vi "serialization tests.vi"() -> ()   [LabVIEW 2013, in "TEC tests.lvlib"]
uses:
  TEC tests.lvlib
  <vilib>/NI/Tag Bus Module Framework/channel/channel classification.ctl
  configuration/TEC configuration.lvclass
  <vilib>/NI/Configuration Framework/serializable configuration/NISE_CEF_serializable configuration.lvclass/NISE_CEF_serializable configuration.ctl
  <vilib>/NI/Configuration Framework/serializable configuration/NISE_CEF_serializable configuration.lvclass
  configuration/TEC configuration.lvclass/TEC configuration.ctl
  <vilib>/NI/Configuration Framework/serializable configuration/Read UID.vi
  configuration/Write channels.vi
  configuration/Read channels.vi
  <vilib>/NI/Tag Bus Module Framework/channel/TBM channel.lvclass
panel:
  out "channels equal":bool
  out "no error":errorcluster
  out "no error":errorcluster
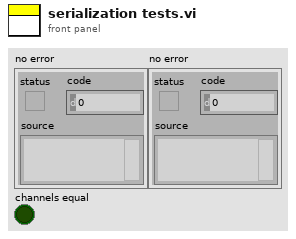
[diagram p1: front panel]
types:
  T1 = typedef "TBM channel.lvclass/channel classification.ctl" = enum16{"input data", "output data", "processing parameter", "processing result"}
  T2 = typedef "tag bus.lvlib/tag descriptor.lvclass/Data Type.ctl" = enum16{"Double", "Single", "I64", "I32", "I16", "I8", "U64", "U32", "U16", "U8", "Boolean", "String", "Array of Double", "Array of Single", "Array of I64", "Array of I32", "Array of I16", "Array of I8", "Array of U64", "Array of U32", "Array of U16", "Array of U8", "Array of Boolean", "Array of String"}
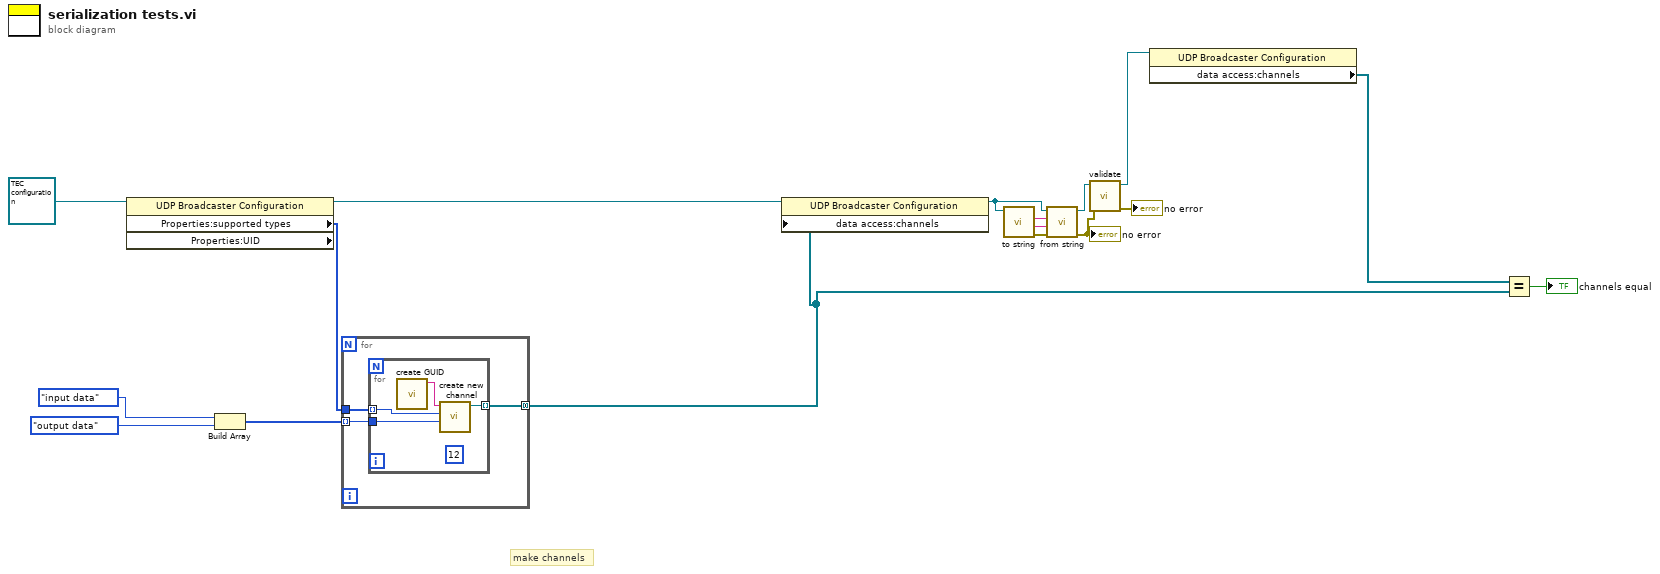
[diagram p0: block diagram]
diagram:
  # "make channels"
  n1 = property class="UDP Broadcaster Configuration" props=["Properties:supported types", "Properties:UID"](reference=refnum<class "TEC configuration.lvclass"> refnum ("tag bus configurable plugin module configuration")) -> (reference out=w5:refnum<class "TEC configuration.lvclass">, "Properties:supported types"=w9:T2[])  [unwired: 1 in, 2 out]
  n2 = Build Array(channel_classification."input data" ("channel classification"), channel_classification."output data" ("channel classification")) -> (w10:T1[])
  n3 = for {
    tunnel: w10 -> [w20] mode=indexing
    tunnel: [w19] -> w1 mode=concatenating
    tunnel: w9 -> [w18]
    n4 = for {
      tunnel: w20 -> [w23]
      tunnel: [w24] -> w19 mode=indexing
      tunnel: w18 -> [w22] mode=indexing
      (unwired) 12
      n5 = call <vilib>:"create GUID.vi"() -> ("uuid"=w21:string)  [unwired: 11 in]
      n6 = call <vilib>:"create new channel.vi"("channel classification"=w23, "data type"=w22, "channel name"=w21) -> ("channel"=w24:refnum<class "TBM channel.lvclass">)  [unwired: 8 in]
    }
  }
  n7 = property class="UDP Broadcaster Configuration"(reference=w5, "data access:channels"=w1) -> (reference out=w2:refnum<class "TEC configuration.lvclass">)  [unwired: 1 in, 1 out]
  n8 = call-dynamic "to string.vi"("TEC configuration in"=w2) -> ("error out"=w17:errorcluster, "data"=w16:string, "version"=w15:string)  [unwired: 7 in, 1 out]
  n9 = call-dynamic "from string.vi"("error in"=w17, "data"=w16, "version"=w15, "TEC configuration in"=w2) -> ("error out"=w8:errorcluster, "TEC configuration out"=w14:refnum<class "TEC configuration.lvclass">)  [unwired: 6 in]
  "no error" <- w8
  n10 = call-dynamic "validate.vi"("error in"=w8, "TEC configuration in"=w14) -> ("error out"=→"no error":errorcluster, "TEC configuration out"=w4:refnum<class "TEC configuration.lvclass">)  [unwired: 8 in]
  n11 = property class="UDP Broadcaster Configuration"(reference=w4) -> ("data access:channels"=w3:refnum<class "TBM channel.lvclass">[])  [unwired: 1 in, 2 out]
  n12 = Equal?(x=w3, y=w1) -> (x = y?=→"channels equal":bool)
